vi "ast_reql_cache.vi"(7 "action":T1, 10 "query in":string, 11 "reql_id in":u32 format="%08x") -> (1 "exists?":bool, 2 "query out":string, 3 "reql_id out":u32 format="%08x")   [LabVIEW 2017]
uses:
  ast_reql_cache_action.ctl
panel:
  out "reql_ids":u32[](array[numeric]) format="%08x"
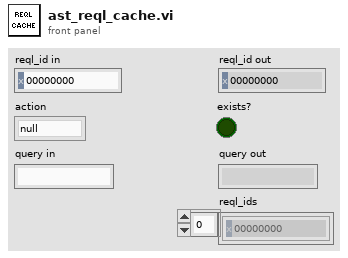
[diagram p1: front panel]
types:
  T1 = typedef "ast_reql_cache_action.ctl" = enum8{"null", "new", "get_query", "get_response", "set_query", "set_response", "delete"}
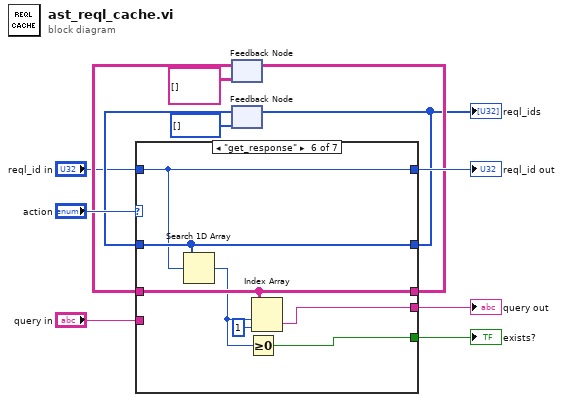
[diagram p0: block diagram]
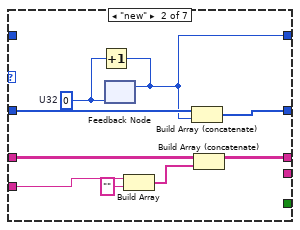
[diagram p3: hidden frame]
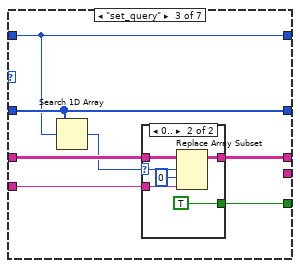
[diagram p4: hidden frame]
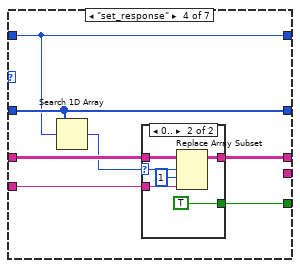
[diagram p6: hidden frame]
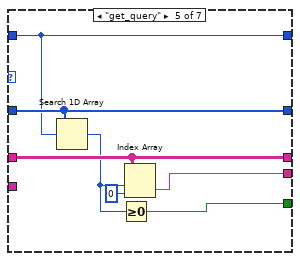
[diagram p8: hidden frame]
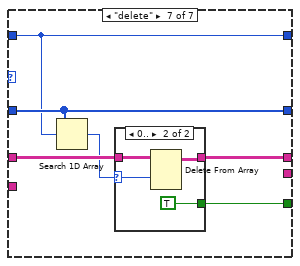
[diagram p9: hidden frame]
diagram:
  n1 = feedback #1(string[][] []) -> (w6:string[][])
  n2 = feedback #2(u32[] []) -> (w8:u32[])
  n3 = case shown="\"get_response\"" "action" {
    tunnel: [w13 w19 w30 w44 w58 w65 w71] -> w12
    tunnel: w8 -> [w15 w24 w31 w45 w59 w66 w72]
    tunnel: [w15 w23 w31 w45 w59 w66 w72] -> w1
    tunnel: [w14 w21 w28 w42 w57 w64 w68] -> w7
    tunnel: w6 -> [w14 w22 w29 w43 w57 w64 w70]
    tunnel: "reql_id in" -> [w13 _ w30 w44 w58 w65 w71]
    tunnel: "query in" -> [_ w18 w26 w40 _ _ _]
    tunnel: [_ _ _ _ w56 w63 _] -> w3
    tunnel: [_ _ w25 w39 w54 w61 w67] -> w2
    frame "null" {
    }
    frame "new" {
      w20 = u32 0  # U32
      n4 = Increment(x=w20) -> (x+1=w19:u32)
      n5 = feedback #3(w20) -> ()  [unwired: 1 in]
      n6 = feedback-in #3(w19) -> ()
      n7 = Build Array(w18, "" ("element")) -> (w17:string[])
      n8 = Build Array (concatenate)(w24, w19) -> (w23:u32[])
      n9 = Build Array (concatenate)(w22, w17) -> (w21:string[][])
    }
    frame "set_query" {
      n10 = Search 1D Array(1D array=w31, element=w30) -> (index of element=w27:i32)  [unwired: 1 in]
      n11 = case shown="0.." w27 {
        selector: w27 -> [_ w36]
        tunnel: w29 -> [w32 w38]
        tunnel: [w32 w37] -> w28
        tunnel: w26 -> [_ w35]
        tunnel: [_ TRUE] -> w25
        frame ..-1 {
        }
        frame 0.. {
          n12 = Replace Array Subset(array=w38, new element=w35, index (row)=w36, index (col)=0 ("disabled index (col)")) -> (w37:string[][])
        }
      }
    }
    frame "set_response" {
      n13 = Search 1D Array(1D array=w45, element=w44) -> (index of element=w41:i32)  [unwired: 1 in]
      n14 = case shown="0.." w41 {
        selector: w41 -> [_ w50]
        tunnel: w43 -> [w46 w52]
        tunnel: [w46 w51] -> w42
        tunnel: w40 -> [_ w49]
        tunnel: [_ TRUE] -> w39
        frame ..-1 {
        }
        frame 0.. {
          n15 = Replace Array Subset(array=w52, new element=w49, index (row)=w50, index (col)=1 ("disabled index (col)")) -> (w51:string[][])
        }
      }
    }
    frame "get_query" {
      n16 = Search 1D Array(1D array=w59, element=w58) -> (index of element=w55:i32)  [unwired: 1 in]
      n17 = Greater Or Equal To 0?(x=w55) -> (x >= 0?=w54:bool)
      n18 = Index Array(array=w57, index (row)=w55, index (col)=0 ("disabled index (col)")) -> (element=w56:string)
    }
    frame "get_response" {
      n19 = Search 1D Array(1D array=w66, element=w65) -> (index of element=w62:i32)  [unwired: 1 in]
      n20 = Greater Or Equal To 0?(x=w62) -> (x >= 0?=w61:bool)
      n21 = Index Array(array=w64, index (row)=w62, index (col)=1 ("disabled index (col)")) -> (element=w63:string)
    }
    frame "delete" {
      n22 = Search 1D Array(1D array=w72, element=w71) -> (index of element=w69:i32)  [unwired: 1 in]
      n23 = case shown="0.." w69 {
        selector: w69 -> [_ w76]
        tunnel: w70 -> [w73 w77]
        tunnel: [w73 w75] -> w68
        tunnel: [_ TRUE] -> w67
        frame ..-1 {
        }
        frame 0.. {
          n24 = Delete From Array(array=w77, index (row)=w76) -> (array with subset deleted=w75:string[][])  [unwired: 2 in, 1 out]
        }
      }
    }
  }
  "reql_id out" <- w12
  "query out" <- w3
  "exists?" <- w2
  "reql_ids" <- w1
  n25 = feedback-in #1(w7) -> ()
  n26 = feedback-in #2(w1) -> ()
